vi "Update H.vi"(8 "error in (no error)":errorcluster, 10 "SLAM In":T3, 11 "New LM's In":T2(array[cluster])) -> (0 "error out":errorcluster, 2 "SLAM Out":T3, 3 "New LM's Out":T2(array[cluster]))   [LabVIEW 2009]
uses:
  <vilib>/Analysis/Matrix/Datatypes/RealMatrix.ctl
  Controls/SLAM.ctl
  <vilib>/Analysis/Matrix/NI_Matrix.lvlib
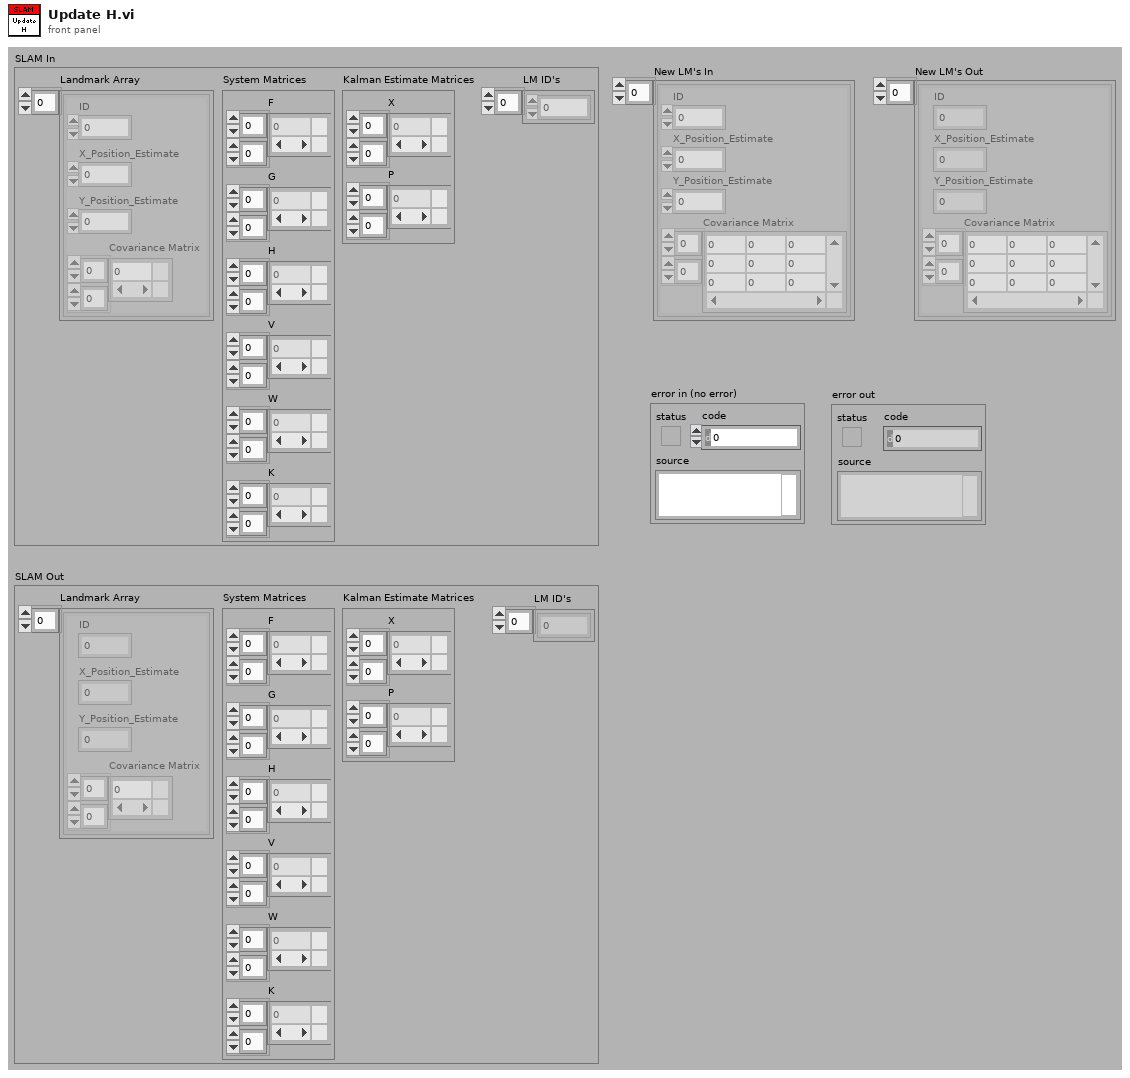
[diagram p1: front panel]
types:
  T1 = typedef "NI_Matrix.lvlib/RealMatrix.ctl" = dbl[][]
  T2 = cluster{"ID":dbl, "X_Position_Estimate":dbl, "Y_Position_Estimate":dbl, "Covariance Matrix":T1}[]
  T3 = typedef "SLAM.ctl" = cluster{"Landmark Array":cluster{"ID":dbl, "X_Position_Estimate":dbl, "Y_Position_Estimate":dbl, "Covariance Matrix":T1}[], "System Matrices":cluster{"F":T1, "G":T1, "H":T1, "V":T1, "W":T1, "K":T1}, "Kalman Estimate Matrices":cluster{"X":T1, "P":T1}, "LM ID's":dbl[]}
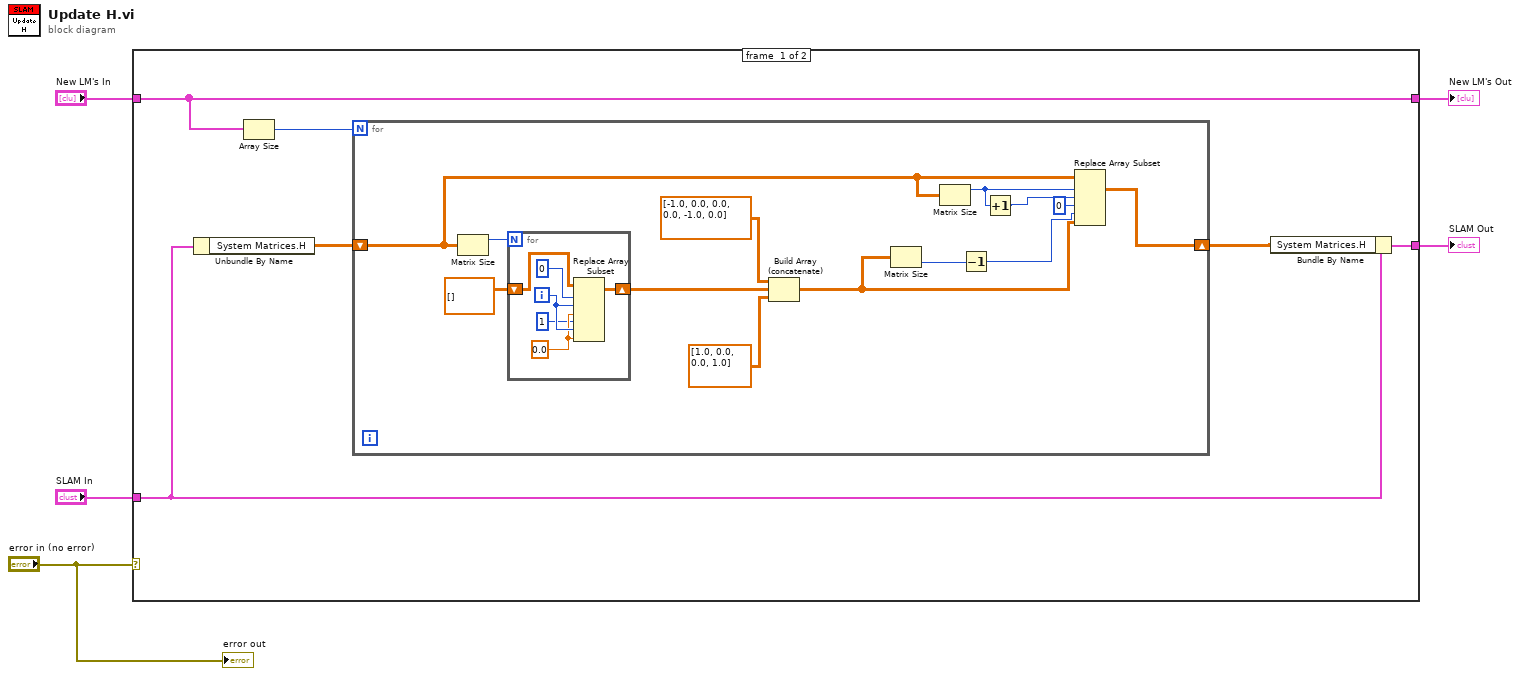
[diagram p0: block diagram]
diagram:
  n1 = case shown="Error" "error in (no error)" {
    tunnel: "SLAM In" -> [w11 w31]
    tunnel: "New LM's In" -> [w9 w32]
    tunnel: [w10 w31] -> w3
    tunnel: [w9 w32] -> w2
    frame #0 {
      n2 = Unbundle By Name(w11) -> ("System Matrices.H"=w8:T1)
      n3 = Array Size(array=w9) -> (size(s)=w7:i32)
      n4 = for {
        N: w7 -> [_]
        shift-right: [w12] -> w6
        shift-left: w8 -> [w13]
        n5 = Matrix Size(0:w13) -> (1:w23:i32)  [unwired: 1 out]
        n6 = for {
          N: w23 -> [_]
          shift-right: [w27] -> w20
          shift-left: T1 [] ("H In") -> [w30]
          i -> [w29]
          w28 = 0.0 ("new element/submatrix")
          n7 = Replace Array Subset(array=w30, new element #1=w28, index (row) #1=0 ("disabled index (row)"), index (col) #1=w29, new element #2=w28, index (row) #2=1 ("disabled index (row)"), index (col) #2=w29) -> (w27:T1)
        }
        n8 = Build Array (concatenate)(T1 [[-1.0, 0.0, 0.0], [0.0, -1.0, 0.0]] ("H In"), w20, T1 [[1.0, 0.0], [0.0, 1.0]] ("H In")) -> (w18:T1)
        n9 = Matrix Size(0:w18) -> (2:w17:i32)  [unwired: 1 out]
        n10 = Matrix Size(0:w13) -> (1:w15:i32)  [unwired: 1 out]
        n11 = Decrement(x=w17) -> (x-1=w16:i32)
        n12 = Increment(x=w15) -> (x+1=w14:i32)
        n13 = Replace Array Subset(array=w13, new element=w18, index (dim 0)=w15, index (dim 1)=w14, index (dim 2)=0 ("column 1"), index (dim 3)=w16) -> (w12:T1)
      }
      n14 = Bundle By Name(cluster=w11, "System Matrices.H"=w6) -> (w10:T3)
    }
    frame #1 {
    }
  }
  "New LM's Out" <- w2
  "SLAM Out" <- w3
  "error out" <- "error in (no error)"
